vi "stage_move_absolute.vi"(7 "Stage Name":string, 8 "error in (no error)":errorcluster, 9 "wait_for_done":bool, 10 "Position":dbl, 11 "Stage in":refnum<class "thorlabs_kinesis.lvclass">) -> (0 "error out":errorcluster, 3 "Stage out":refnum<class "thorlabs_kinesis.lvclass">)   [LabVIEW 2015, in "thorlabs_kinesis.lvclass"]
uses:
  thorlabs_kinesis.lvclass
  thorlabs_kinesis.lvclass/thorlabs_kinesis.ctl
  thorlabs_drivers/Thorlabs.MotionControl.Benchtop.Piezo.dll
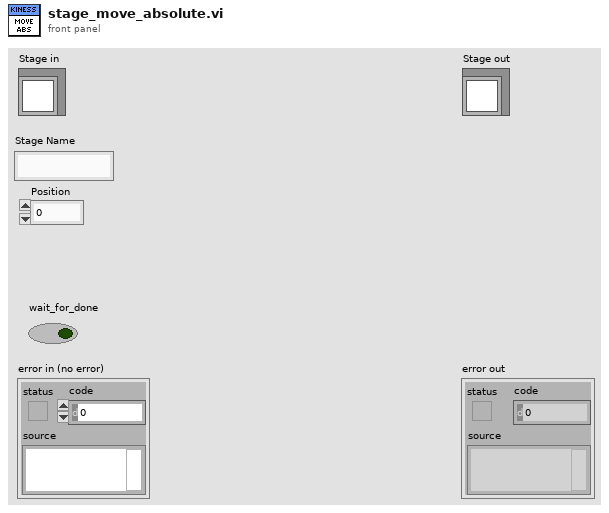
[diagram p1: front panel]
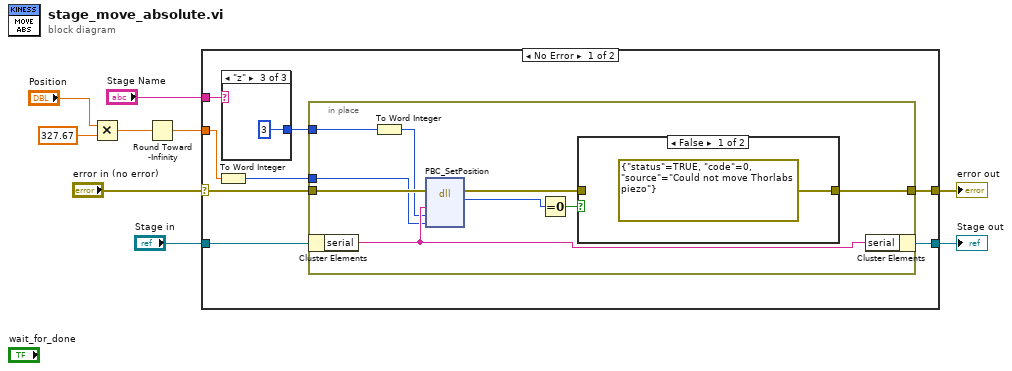
[diagram p0: block diagram]
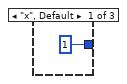
[diagram p2: hidden frame]
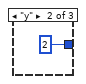
[diagram p3: hidden frame]
diagram:
  n1 = Multiply(x="Position", y=327.67) -> (x*y=w1:dbl)
  n2 = Round Toward -Infinity(1:w1) -> (0:w4:dbl)
  n3 = case shown="No Error" "error in (no error)" {
    selector: "error in (no error)" -> [w15 w33]
    tunnel: [w12 w33] -> w8
    tunnel: [w16 w32] -> w6
    tunnel: "Stage in" -> [w17 w32]
    tunnel: "Stage Name" -> [w11 _]
    tunnel: w4 -> [w14 _]
    frame No Error {
      n4 = To Word Integer(number=w14) -> (16bit integer=w13:i16)
      n5 = case shown="\"z\"" w11 {
        tunnel: [1 2 3] -> w10
        frame "x", Default {
        }
        frame "y" {
        }
        frame "z" {
        }
      }
      n6 = in-place {
        in-place-border: w10 -> [w22]
        in-place-border: w15 -> [w28]
        in-place-border: w13 -> [w27]
        in-place-border: [w23] -> w12
        n7 = in-place-cluster #1(w17) -> ("serial"=w29:string)
        n8 = To Word Integer(number=w22) -> (16bit integer=w21:i16)
        n9 = dll-call lib="C:/Users/MX-Microscope/Documents/LabVIEW Data/lvoop_campus_2018/Stage Class/Thorlabs Kinesis/thorlabs_drivers/Thorlabs.MotionControl.Benchtop.Piezo.dll" fn="PBC_SetPosition"(error in=w28, "serial"=w29, "channel"=w21, "volts"=w27) -> (error out=w24:errorcluster, "return type"=w26:i16)  [unwired: 5 in, 1 out]
        n10 = Equal To 0?(x=w26) -> (x = 0?=w25:bool)
        n11 = case shown="False" w25 {
          tunnel: w24 -> [_ w31]
          tunnel: [errorcluster {"status"=TRUE, "code"=0, "source"="Could not move Thorlabs piezo"} ("error out") w31] -> w23
          frame False {
          }
          frame True {
          }
        }
        n12 = in-place-cluster #1("serial"=w29) -> (w16:refnum<class "thorlabs_kinesis.lvclass">)
      }
    }
    frame Error {
    }
  }
  "error out" <- w8
  "Stage out" <- w6
